vi "_FPGA_Counting_U8.vi"(1 "Reset":bool, 2 "Increase":bool) -> (0 "Num out":u8)   [LabVIEW 2018]
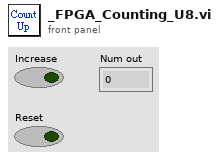
[diagram p1: front panel]
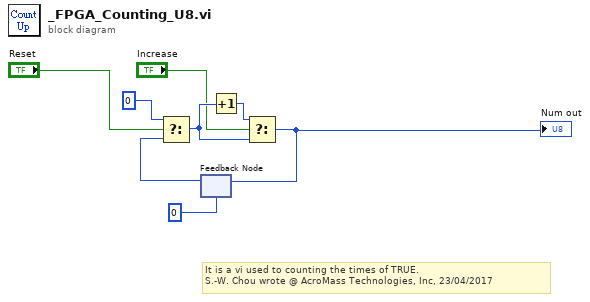
[diagram p0: block diagram]
diagram:
  # "It is a vi used to counting the times of TRUE.\nS.-W. Chou wrote @ AcroMass Technologies, Inc, 23/04/2017"
  n1 = feedback #1(u8 0) -> (w5:u8)
  n2 = Select(t=u8 0, s="Reset", f=w5) -> (s? t:f=w6:u8)
  n3 = Increment(x=w6) -> (x+1=w4:u8)
  n4 = Select(t=w4, s="Increase", f=w6) -> (s? t:f=w7:u8)
  "Num out" <- w7
  n5 = feedback-in #1(w7) -> ()
